vi "Configure Jitter Spectrum Plot Type.vi"(8 "error in (no error)":errorcluster, 10 "Plot Type (0: Linear)":i32(ring) items=["Linear", "Log Arithmic"], 11 "VISA resource name":refnum<visa-resource-name>) -> (0 "error out":errorcluster, 3 "VISA resource name out":refnum<visa-resource-name>)   [LabVIEW 2020, in "Agilent 90000 Series.lvlib"]
doc: "Configures the type for the jitter spectrum plot."
uses:
  Agilent 90000 Series.lvlib
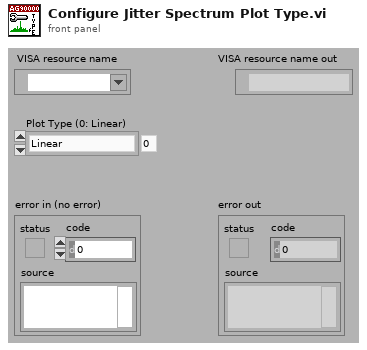
[diagram p1: front panel]
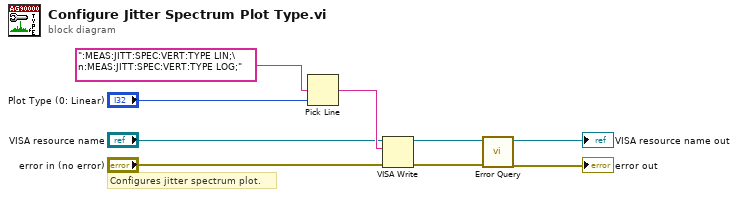
[diagram p0: block diagram]
diagram:
  # "Configures jitter spectrum plot."
  n1 = Pick Line(multi-line string=":MEAS:JITT:SPEC:VERT:TYPE LIN;\n:MEAS:JITT:SPEC:VERT:TYPE LOG;", line index="Plot Type (0: Linear)") -> (output string=w7:string)  [unwired: 1 out]
  n2 = VISA Write(VISA resource name="VISA resource name", write buffer=w7, error in (no error)="error in (no error)") -> (VISA resource name out=w4:refnum<visa-resource-name>, error out=w3:errorcluster)  [unwired: 1 out]
  n3 = call "Error Query.vi"("error in (no error)"=w3, "VISA resource name"=w4) -> ("error out"=→"error out":errorcluster, "VISA resource name out"=→"VISA resource name out":refnum<visa-resource-name>)  [unwired: 8 out]
